vi "EoTDetect.vi"(9 "Loops":i32=10, 10 "Tolerance":dbl=0.1, 11 "Sensor":dbl) -> (3 "EoT? (F)":bool)   [LabVIEW 2014, in "Elevator System.lvlib"]
uses:
  Elevator System.lvlib
  <vilib>/ptbypt/NI_PtbyPt.lvlib
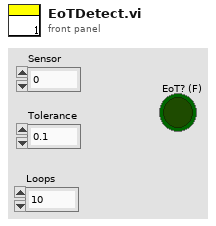
[diagram p1: front panel]
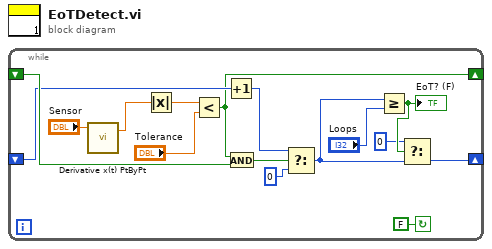
[diagram p0: block diagram]
diagram:
  n1 = while {
    shift-right: [w6] -> _
    shift-left: _ -> [w14]
    shift-right: [w3] -> _
    shift-left: _ -> [w11]
    stop <- FALSE continue-if-true
    n2 = call <vilib>:"Derivative x(t) PtByPt.vi"("x"="Sensor") -> ("dx/dt"=w5:dbl)  [unwired: 3 in, 1 out]
    n3 = Absolute Value(x=w5) -> (abs(x)=w15:dbl)
    n4 = Less?(x=w15, y="Tolerance") -> (x < y?=w6:bool)
    n5 = Increment(x=w11) -> (x+1=w10:i32)
    n6 = And(x=w6, y=w14) -> (x .and. y?=w13:bool)
    n7 = Select(t=w10, s=w13, f=0) -> (s? t:f=w7:i32)
    n8 = Greater Or Equal?(x=w7, y="Loops") -> (x >= y?=w2:bool)
    "EoT? (F)" <- w2
    n9 = Select(t=0, s=w2, f=w7) -> (s? t:f=w3:i32)
  }
